vi "dfd_DFXP_Decimal Length Difference.vi"(8 "iwl 2":i16, 9 "wl 2":i16, 10 "iwl 1":i16, 11 "wl 1":i16) -> (0 "fwl_diff <= 0?":bool, 1 "fwl_diff":i16, 2 "fwl":i16, 3 "iwl_diff >= 0?":bool, 5 "iwl_diff >= 64?":bool)   [LabVIEW 2017, in "NI_DigFilter_FXP.lvlib"]
uses:
  <vilib>/addons/Digital Filter Design/NI_DigFilter_FXP.lvlib
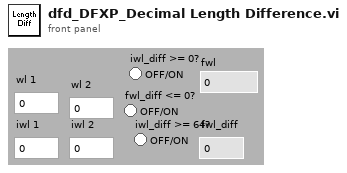
[diagram p1: front panel]
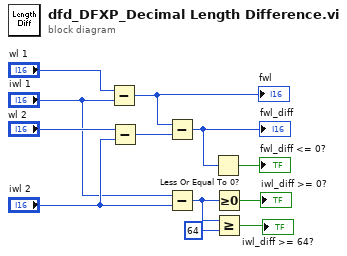
[diagram p0: block diagram]
diagram:
  n1 = Subtract(x="wl 1", y="iwl 1") -> (x-y=w4:i16)
  "fwl" <- w4
  n2 = Subtract(x="wl 2", y="iwl 2") -> (x-y=w6:i16)
  n3 = Subtract(x=w4, y=w6) -> (x-y=w10:i16)
  "fwl_diff" <- w10
  n4 = Subtract(x="iwl 1", y="iwl 2") -> (x-y=w3:i16)
  n5 = Less Or Equal To 0?(x=w10) -> (x <= 0?=→"fwl_diff <= 0?":bool)
  n6 = Greater Or Equal To 0?(x=w3) -> (x >= 0?=→"iwl_diff >= 0?":bool)
  n7 = Greater Or Equal?(x=w3, y=i16 64) -> (x >= y?=→"iwl_diff >= 64?":bool)
